vi "Register Pin Map.vi"(8 "error in":errorcluster, 11 "pin map file path":path) -> (0 "error out":errorcluster, 3 "pin map id":string)   [LabVIEW 2021, in "NI Pin Map V1 Client.lvlib"]
doc: "Registers given pin map with the pin map service."
uses:
  NI Pin Map V1 Client.lvlib
  gRPC/Generated APIs/ni/measurementlink/pinmap/v1/RPC Messages/ni_measurementlink_pinmap_v1_UpdatePinMapFromXmlRequest.ctl
  gRPC/Generated APIs/ni/measurementlink/pinmap/v1/ni.measurementlink.pinmap.v1.api.lvlib
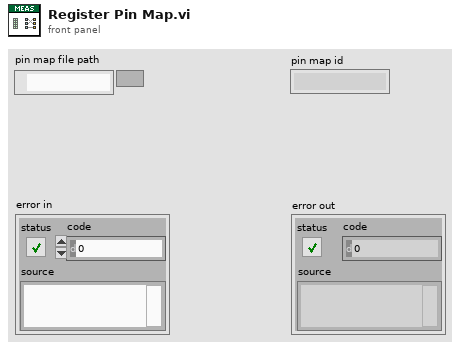
[diagram p1: front panel]
types:
  T1 = typedef "ni.measurementlink.pinmap.v1.api.lvlib/ni_measurementlink_pinmap_v1_UpdatePinMapFromXmlRequest.ctl" = cluster{"pin_map_id":string, "pin_map_xml":string}
  T2 = typedef "ni.measurementlink.pinmap.v1.api.lvlib/ni_measurementlink_pinmap_v1_PinMap.ctl" = cluster{"pin_map_id":string}
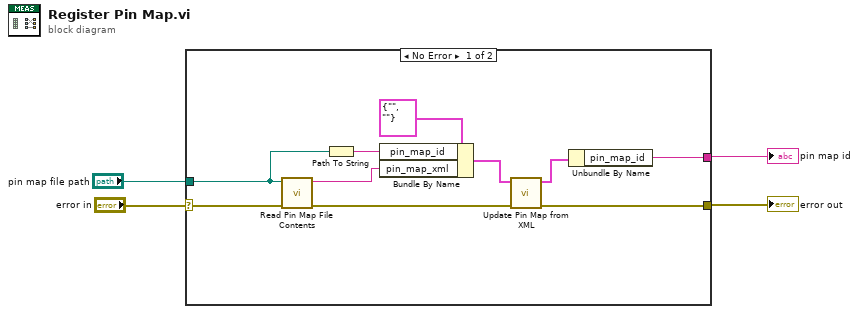
[diagram p0: block diagram]
diagram:
  n1 = case shown="No Error" "error in" {
    selector: "error in" -> [w14 w15]
    tunnel: [w9 w15] -> w1
    tunnel: "pin map file path" -> [w6 _]
    tunnel: [w5 _] -> w2
    frame No Error {
      n2 = call "Read Pin Map File Contents.vi"("error in"=w14, "pin map file path"=w6) -> ("error out"=w13:errorcluster, "pin map xml"=w7:string)  [unwired: 8 in]
      n3 = Path To String(path=w6) -> (string=w12:string)
      n4 = Bundle By Name(cluster=T1 {"pin_map_id"="", "pin_map_xml"=""} ("request data"), "pin_map_id"=w12, "pin_map_xml"=w7) -> (w10:T1)
      n5 = call "Update Pin Map from XML.vi"("error in"=w13, "request data"=w10) -> ("error out"=w9:errorcluster, "response data"=w8:T2)  [unwired: 8 in]
      n6 = Unbundle By Name(w8) -> ("pin_map_id"=w5:string)
    }
    frame Error {
    }
  }
  "pin map id" <- w2
  "error out" <- w1
